vi "2~100条码ID.vi"(10 "MES配置输入":T2, 11 "条码字符串输入":T1) -> (1 "时间":string, 2 "MES字符串":string, 3 "1-99":string)   [LabVIEW 2014]
panel:
  in  "字符串":string
  out "匹配子字符串":string
  in  "工位1字符串":string
  in  "工位2字符串":string
  out "数组":string[](array[string])
  out "数组 2":string[](array[string])
  out "日期字符串":string
  out "时间字符串":string
  out "56~100":string[](array[string])
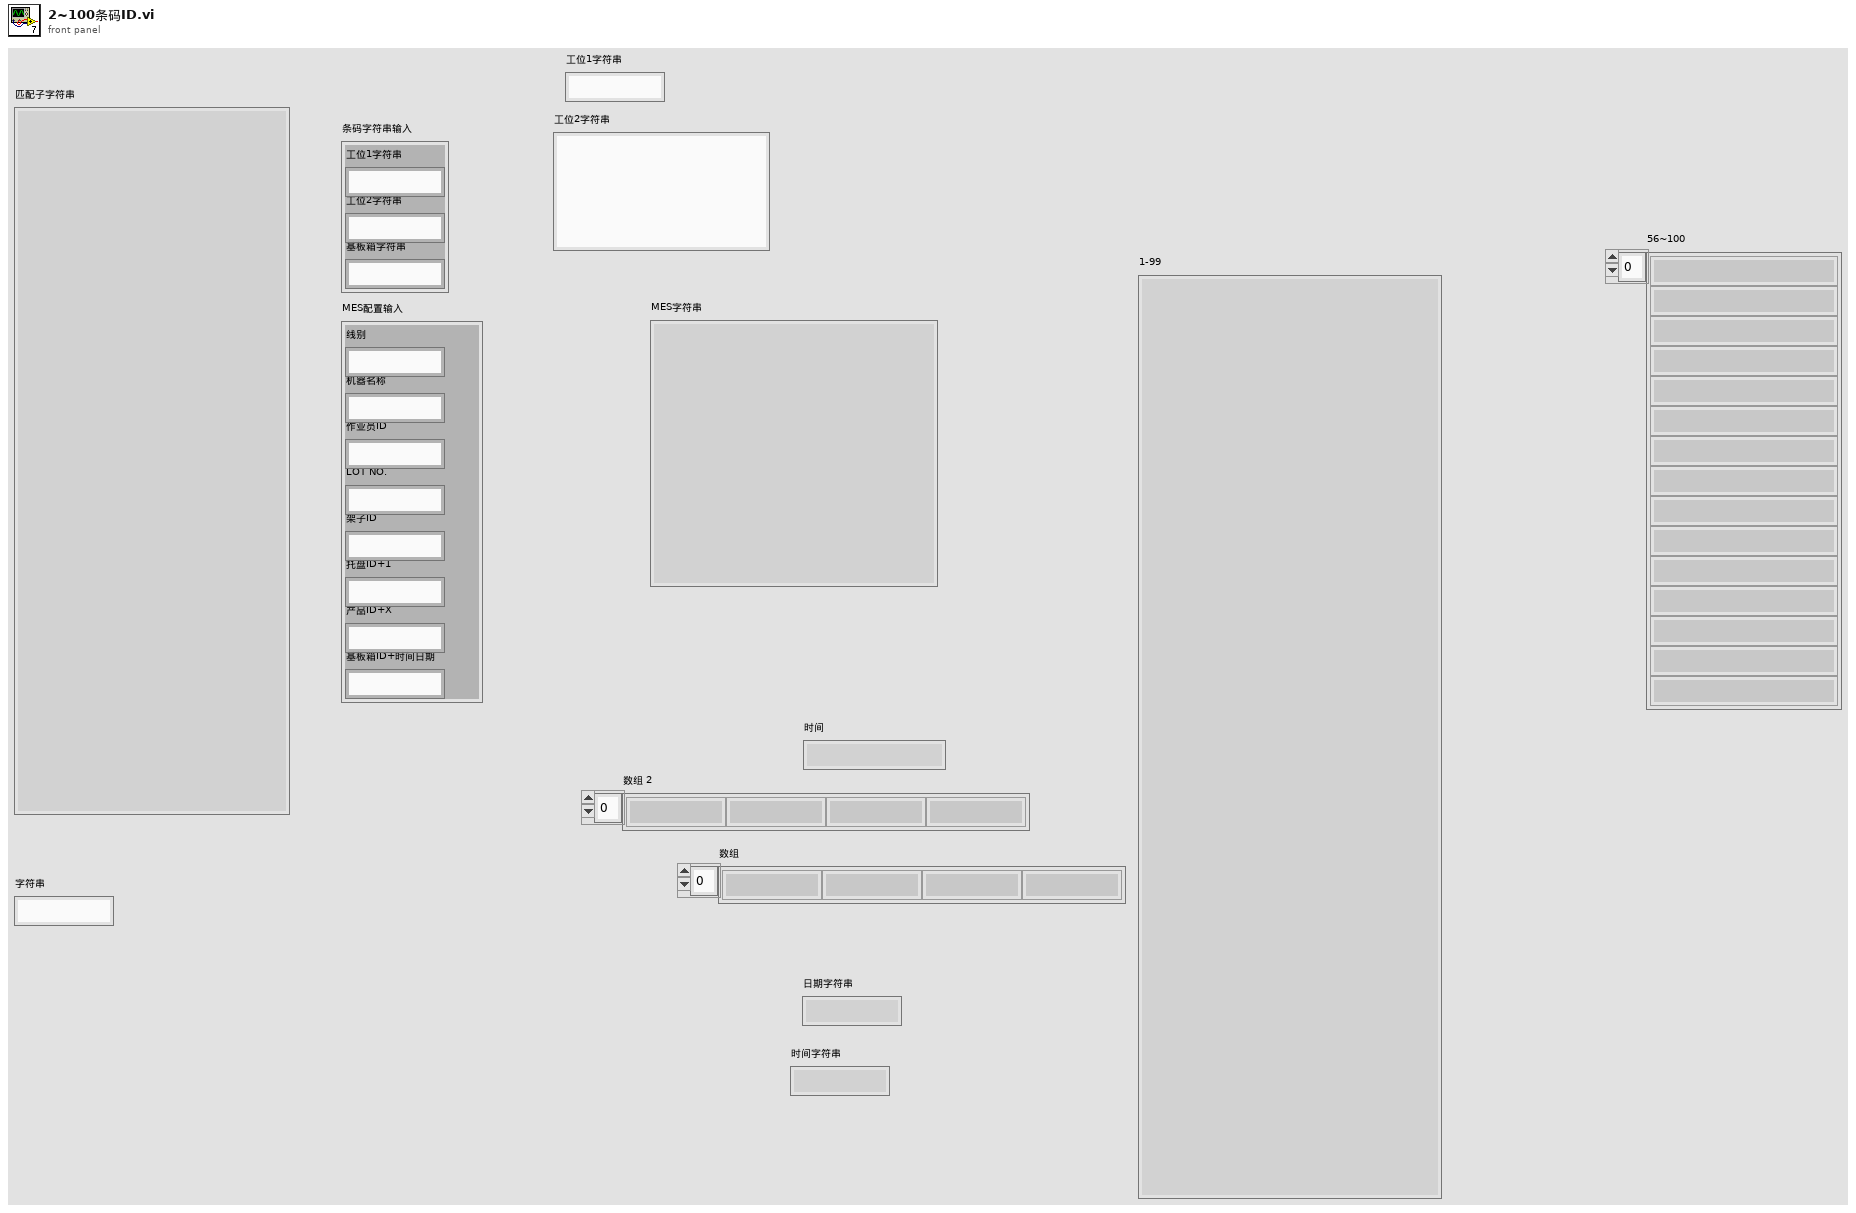
[diagram p1: front panel]
types:
  T1 = cluster{"工位1字符串":string, "工位2字符串":string, "基板箱字符串":string}
  T2 = cluster{"线别":string, "机器名称":string, "作业员ID":string, "LOT NO.":string, "架子ID":string, "托盘ID+1":string, "产品ID+X":string, "基板箱ID+时间日期":string}
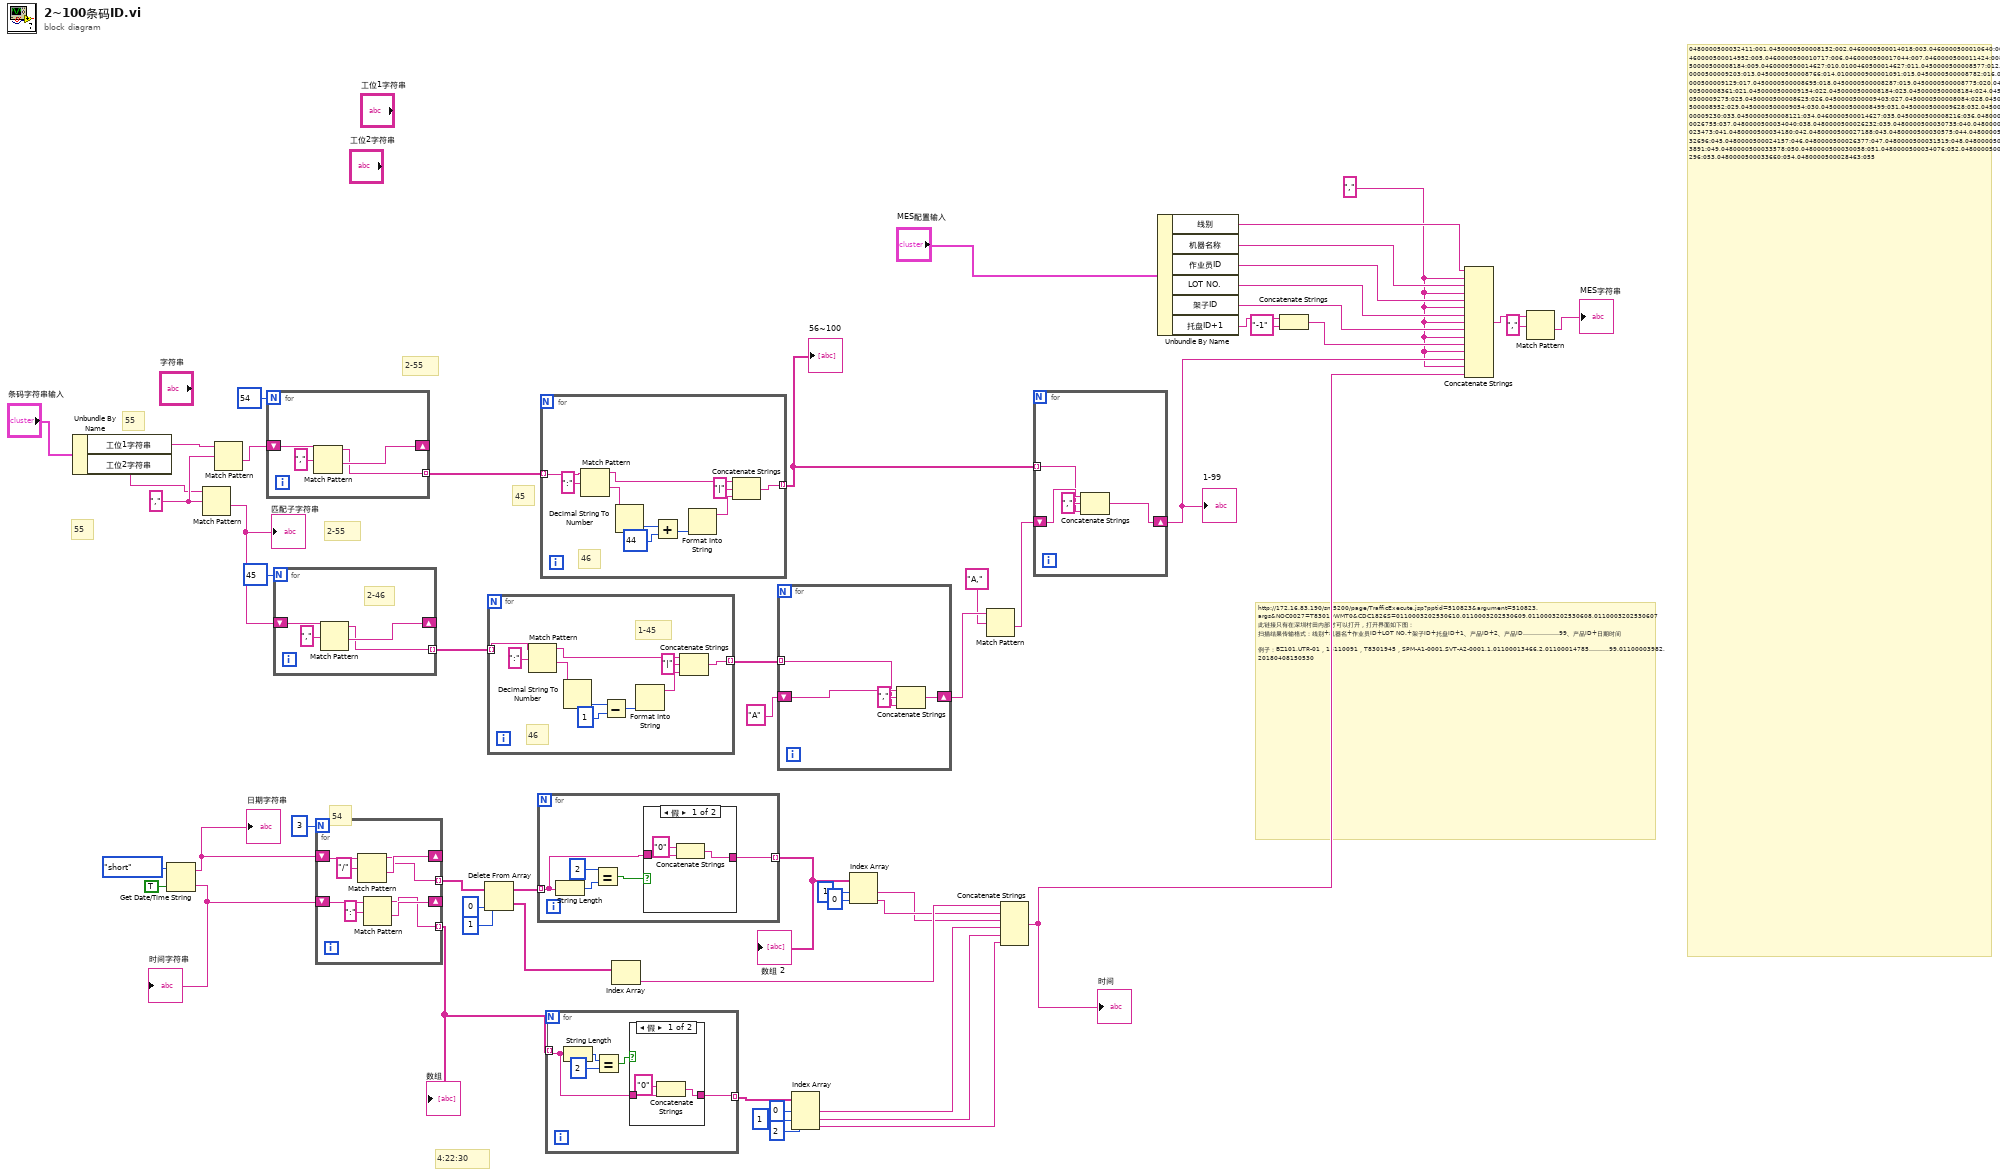
[diagram p0: block diagram]
diagram:
  w13 = "," ("正则表达式")
  w17 = ","
  # "2-55"
  # "2-55"
  # "55"
  # "55"
  # "0480000500032411:001,0450000500008152:002,0460000500014018:003,0460000500010640:004,0460000500014952:005,0460000500010717:006,0460000500017044:007,0460000500011424:008,0450000500008184:009,0460000500014627:010,0100460500014627:011,0450000500008577:012,0450000500009203:013,0450000500008766:014,0100000900001091:015,0450000500008782:016,0450000500009129:017,0450000500008695:018,0450000500008287:019,0450000500008775:020,0450000500008361:021,0450000500009154:022,0450000500008184:023,0450000500008184:024,0450000500009275:025,0450000500008625:026,0450000500009403:027,0450000500008084:028,0450000500008952:029,0450000500009054:030,0450000500008499:031,0450000500009628:032,0450000500009230:033,0450000500008121:034,0460000500014627:035,0450000500008216:036,0480000500026755:037,0480000500034040:038,0480000500026232:039,0480000500030735:040,0480000500023473:041,0480000500034180:042,0480000500027188:043,0480000500030575:044,0480000500032696:045,0480000500024157:046,0480000500026377:047,0480000500031519:048,0480000500023891:049,0480000500033578:050,0480000500030058:051,0480000500034076:052,0480000500023296:053,0480000500033660:054,0480000500028463:055"
  # "4:22:30"
  # "http://172.16.83.190/sm5200/page/TrafficExecute.jsp?pptid=510823&argument=510823.args&NOC0027=T83019WMT0&CDC1826S=0110003202530610,0110003202530609,0110003202530608,0110003202530607\n此链接只有在深圳村田内部才可以打开，打开界面如下图：\n扫描结果传输格式：线别+机器名+作业员ID+LOT NO.+架子ID+托盘ID+1、产品ID+2、产品ID………………99、产品ID+日期时间\n                             例子：BZ101,UTR-01，18110091，T8301945，SPM-A1-0001,SVT-A2-0001,1,01100013466,2,01100014785……….99,01100003982,20180408150530"
  # "54"
  # "45"
  n1 = Unbundle By Name("条码字符串输入") -> ("工位1字符串"=w2:string, "工位2字符串"=w1:string)
  n2 = Get Date/Time String(date format (0)=enum16{"short", "long", "abbreviated"}."short" ("日期格式(0)"), want seconds? (F)=TRUE ("需要秒？(F)")) -> (date string=w43:string, time string=w30:string)  [unwired: 1 in]
  "时间字符串" <- w30
  "日期字符串" <- w43
  n3 = Match Pattern(string=w1, regular expression=w13) -> (after substring=w12:string)  [unwired: 1 in, 3 out]
  "匹配子字符串" <- w12
  n4 = Match Pattern(string=w2, regular expression=w13) -> (after substring=w3:string)  [unwired: 1 in, 3 out]
  n5 = for {
    N: 54 -> [_]
    shift-right: [w57] -> _
    shift-left: w3 -> [w59]
    tunnel: [w56] -> w4 mode=indexing
    n6 = Match Pattern(string=w59, regular expression="," ("正则表达式")) -> (before substring=w56:string, after substring=w57:string)  [unwired: 1 in, 2 out]
  }
  n7 = for {
    N: 45 -> [_]
    shift-right: [w61] -> _
    shift-left: w12 -> [w63]
    tunnel: [w60] -> w10 mode=indexing
    # "2-46"
    n8 = Match Pattern(string=w63, regular expression="," ("正则表达式")) -> (before substring=w60:string, after substring=w61:string)  [unwired: 1 in, 2 out]
  }
  n9 = for {
    N: 3 -> [_]
    shift-right: [w69] -> _
    shift-left: w43 -> [w71]
    tunnel: [w68] -> w41 mode=indexing
    shift-right: [w65] -> _
    shift-left: w30 -> [w67]
    tunnel: [w64] -> w29 mode=indexing
    n10 = Match Pattern(string=w71, regular expression="/" ("正则表达式")) -> (before substring=w68:string, after substring=w69:string)  [unwired: 1 in, 2 out]
    n11 = Match Pattern(string=w67, regular expression=":" ("正则表达式")) -> (before substring=w64:string, after substring=w65:string)  [unwired: 1 in, 2 out]
  }
  "数组" <- w29
  n12 = Delete From Array(array=w41, length=1 ("长度"), index=0 ("索引")) -> (deleted portion=w37:string[], array with subset deleted=w38:string[])
  n13 = for {
    tunnel: w10 -> [w81] mode=indexing
    tunnel: [w77] -> w9 mode=indexing
    # "1-45"
    # "46"
    n14 = Match Pattern(string=w81, regular expression=":" ("正则表达式")) -> (before substring=w79:string, after substring=w78:string)  [unwired: 1 in, 2 out]
    n15 = Decimal String To Number(string=w78) -> (number=w73:i32)  [unwired: 2 in, 1 out]
    n16 = Subtract(x=w73, y=1) -> (x-y=w74:i32)
    n17 = Format Into String(w74) -> (resulting string=w76:string)  [unwired: 3 in, 1 out]
    n18 = Concatenate Strings(w79, "|" ("字符串"), w76) -> (w77:string)
  }
  n19 = for {
    tunnel: w38 -> [w83] mode=indexing
    tunnel: [w82] -> w36 mode=indexing
    n20 = String Length(string=w83) -> (length=w86:i32)
    n21 = Equal?(x=2, y=w86) -> (x = y?=w84:bool)
    n22 = case shown="假" w84 {
      tunnel: w83 -> [w89 w90]
      tunnel: [w87 w90] -> w82
      frame False {
        n23 = Concatenate Strings("0" ("字符串"), w89) -> (w87:string)
      }
      frame True {
      }
    }
  }
  "数组 2" <- w36
  n24 = for {
    tunnel: w4 -> [w100] mode=indexing
    tunnel: [w93] -> w53 mode=indexing
    # "46"
    n25 = Match Pattern(string=w100, regular expression=":" ("正则表达式")) -> (before substring=w98:string, after substring=w97:string)  [unwired: 1 in, 2 out]
    n26 = Decimal String To Number(string=w97) -> (number=w96:i32)  [unwired: 2 in, 1 out]
    n27 = Add(x=w96, y=44) -> (x+y=w94:i32)
    n28 = Format Into String(w94) -> (resulting string=w92:string)  [unwired: 3 in, 1 out]
    n29 = Concatenate Strings(w98, "|" ("字符串"), w92) -> (w93:string)
  }
  "56~100" <- w53
  n30 = for {
    tunnel: w29 -> [w102] mode=indexing
    tunnel: [w101] -> w28 mode=indexing
    n31 = String Length(string=w102) -> (length=w105:i32)
    n32 = Equal?(x=w105, y=2) -> (x = y?=w103:bool)
    n33 = case shown="假" w103 {
      tunnel: w102 -> [w108 w109]
      tunnel: [w107 w109] -> w101
      frame False {
        n34 = Concatenate Strings("0" ("字符串"), w108) -> (w107:string)
      }
      frame True {
      }
    }
  }
  n35 = Index Array(array=w37) -> (element=w33:string)  [unwired: 1 in]
  n36 = for {
    tunnel: w9 -> [w110] mode=indexing
    shift-right: [w113] -> w7
    shift-left: "A" -> [w111]
    n37 = Concatenate Strings(w111, "," ("字符串"), w110) -> (w113:string)
  }
  n38 = Index Array(array=w28, index #1=0 ("索引"), index #2=1 ("索引"), index #3=2 ("索引")) -> (element #1=w24:string, element #2=w23:string, element #3=w22:string)
  n39 = Index Array(array=w36, index #1=1 ("索引"), index #2=0 ("索引")) -> (element #1=w31:string, element #2=w32:string)
  n40 = Match Pattern(string=w7, regular expression="A,") -> (after substring=w5:string)  [unwired: 1 in, 3 out]
  n41 = Concatenate Strings(w33, w32, w31, w24, w23, w22) -> (w21:string)
  "时间" <- w21
  n42 = for {
    tunnel: w53 -> [w114] mode=indexing
    shift-right: [w117] -> w20
    shift-left: w5 -> [w115]
    n43 = Concatenate Strings(w115, "," ("字符串"), w114) -> (w117:string)
  }
  "1-99" <- w20
  n44 = Unbundle By Name("MES配置输入") -> ("线别"=w19:string, "机器名称"=w18:string, "作业员ID"=w49:string, "LOT NO."=w48:string, "架子ID"=w47:string, "托盘ID+1"=w51:string)
  n45 = Concatenate Strings(w51, "-1" ("字符串")) -> (w46:string)
  n46 = Concatenate Strings(w19, w17, w18, w17, w49, w17, w48, w17, w47, w17, w46, w17, w20, w17, w21) -> (w16:string)
  n47 = Match Pattern(string=w16, regular expression="," ("正则表达式")) -> (after substring=→"MES字符串":string)  [unwired: 1 in, 3 out]
